vi "Arduino read multiple frequencies cristains filter.vi"(7 "main loop iteration number":i32, 9 "arduino addresses in":T2, 11 "arduinos on?":bool) -> (1 "arduino addresses out":T2, 2 "arduino frequencies out":T1, 3 "arduinos on":bool)   [LabVIEW 2014]
uses:
  <vilib>/Analysis/baseanly.llb/Mean (DBL).vi
  <vilib>/Analysis/NI_AALBase.lvlib
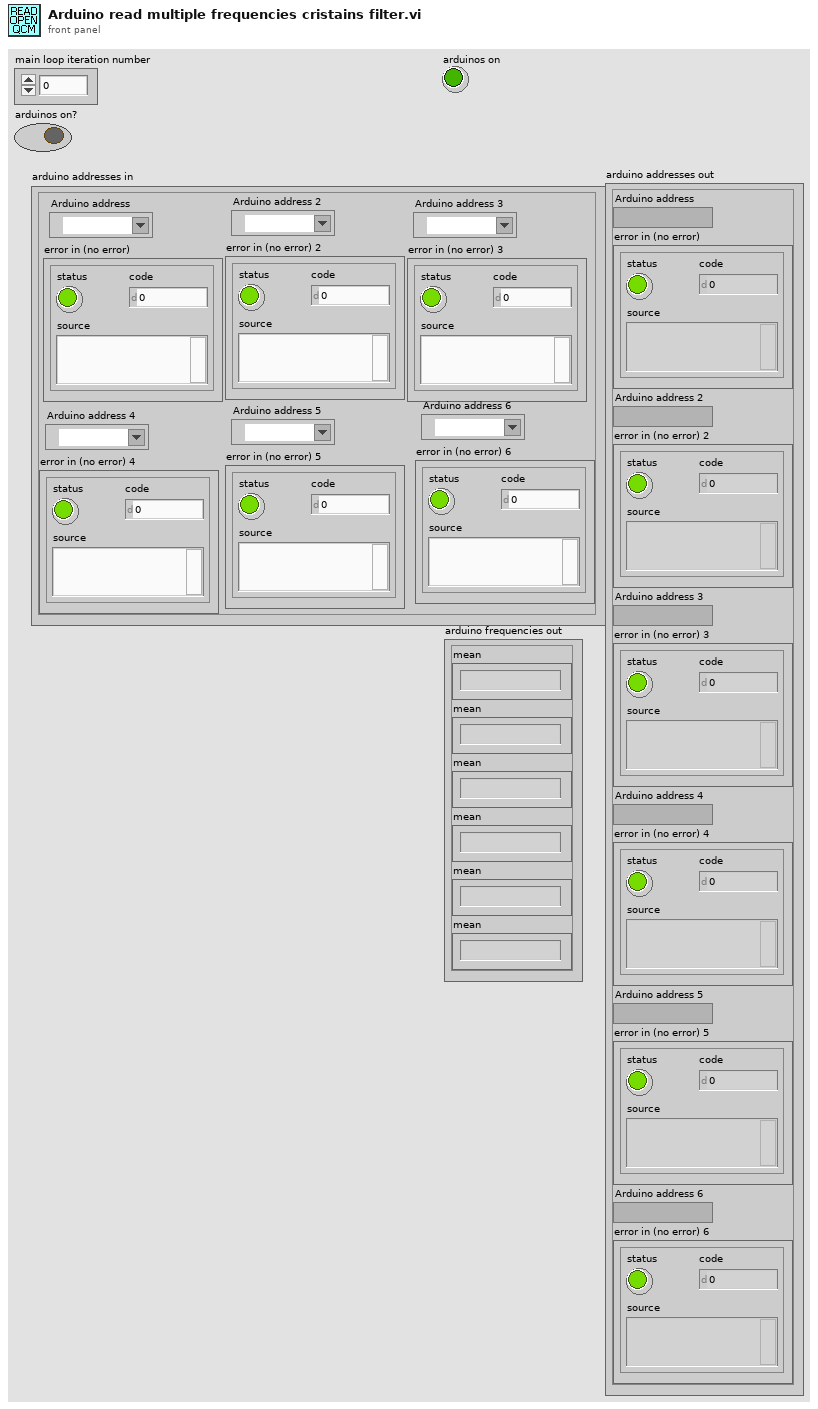
[diagram p1: front panel]
types:
  T1 = cluster{"mean":string, "mean":string, "mean":string, "mean":string, "mean":string, "mean":string}
  T2 = cluster{"Arduino address":refnum<visa-resource-name>, "error in (no error)":errorcluster, "Arduino address 2":refnum<visa-resource-name>, "error in (no error) 2":errorcluster, "Arduino address 3":refnum<visa-resource-name>, "error in (no error) 3":errorcluster, "Arduino address 4":refnum<visa-resource-name>, "error in (no error) 4":errorcluster, "Arduino address 5":refnum<visa-resource-name>, "error in (no error) 5":errorcluster, "Arduino address 6":refnum<visa-resource-name>, "error in (no error) 6":errorcluster}
  T3 = cluster{string, string, string, string, string, string}
  T4 = cluster{"Arduino address":refnum<visa-resource-name>, "error out":errorcluster, "Arduino address 2":refnum<visa-resource-name>, "error out":errorcluster, "Arduino address 3":refnum<visa-resource-name>, "error out":errorcluster, "Arduino address 4":refnum<visa-resource-name>, "error out":errorcluster, "Arduino address 5":refnum<visa-resource-name>, "error out":errorcluster, "Arduino address 6":refnum<visa-resource-name>, "error out":errorcluster}
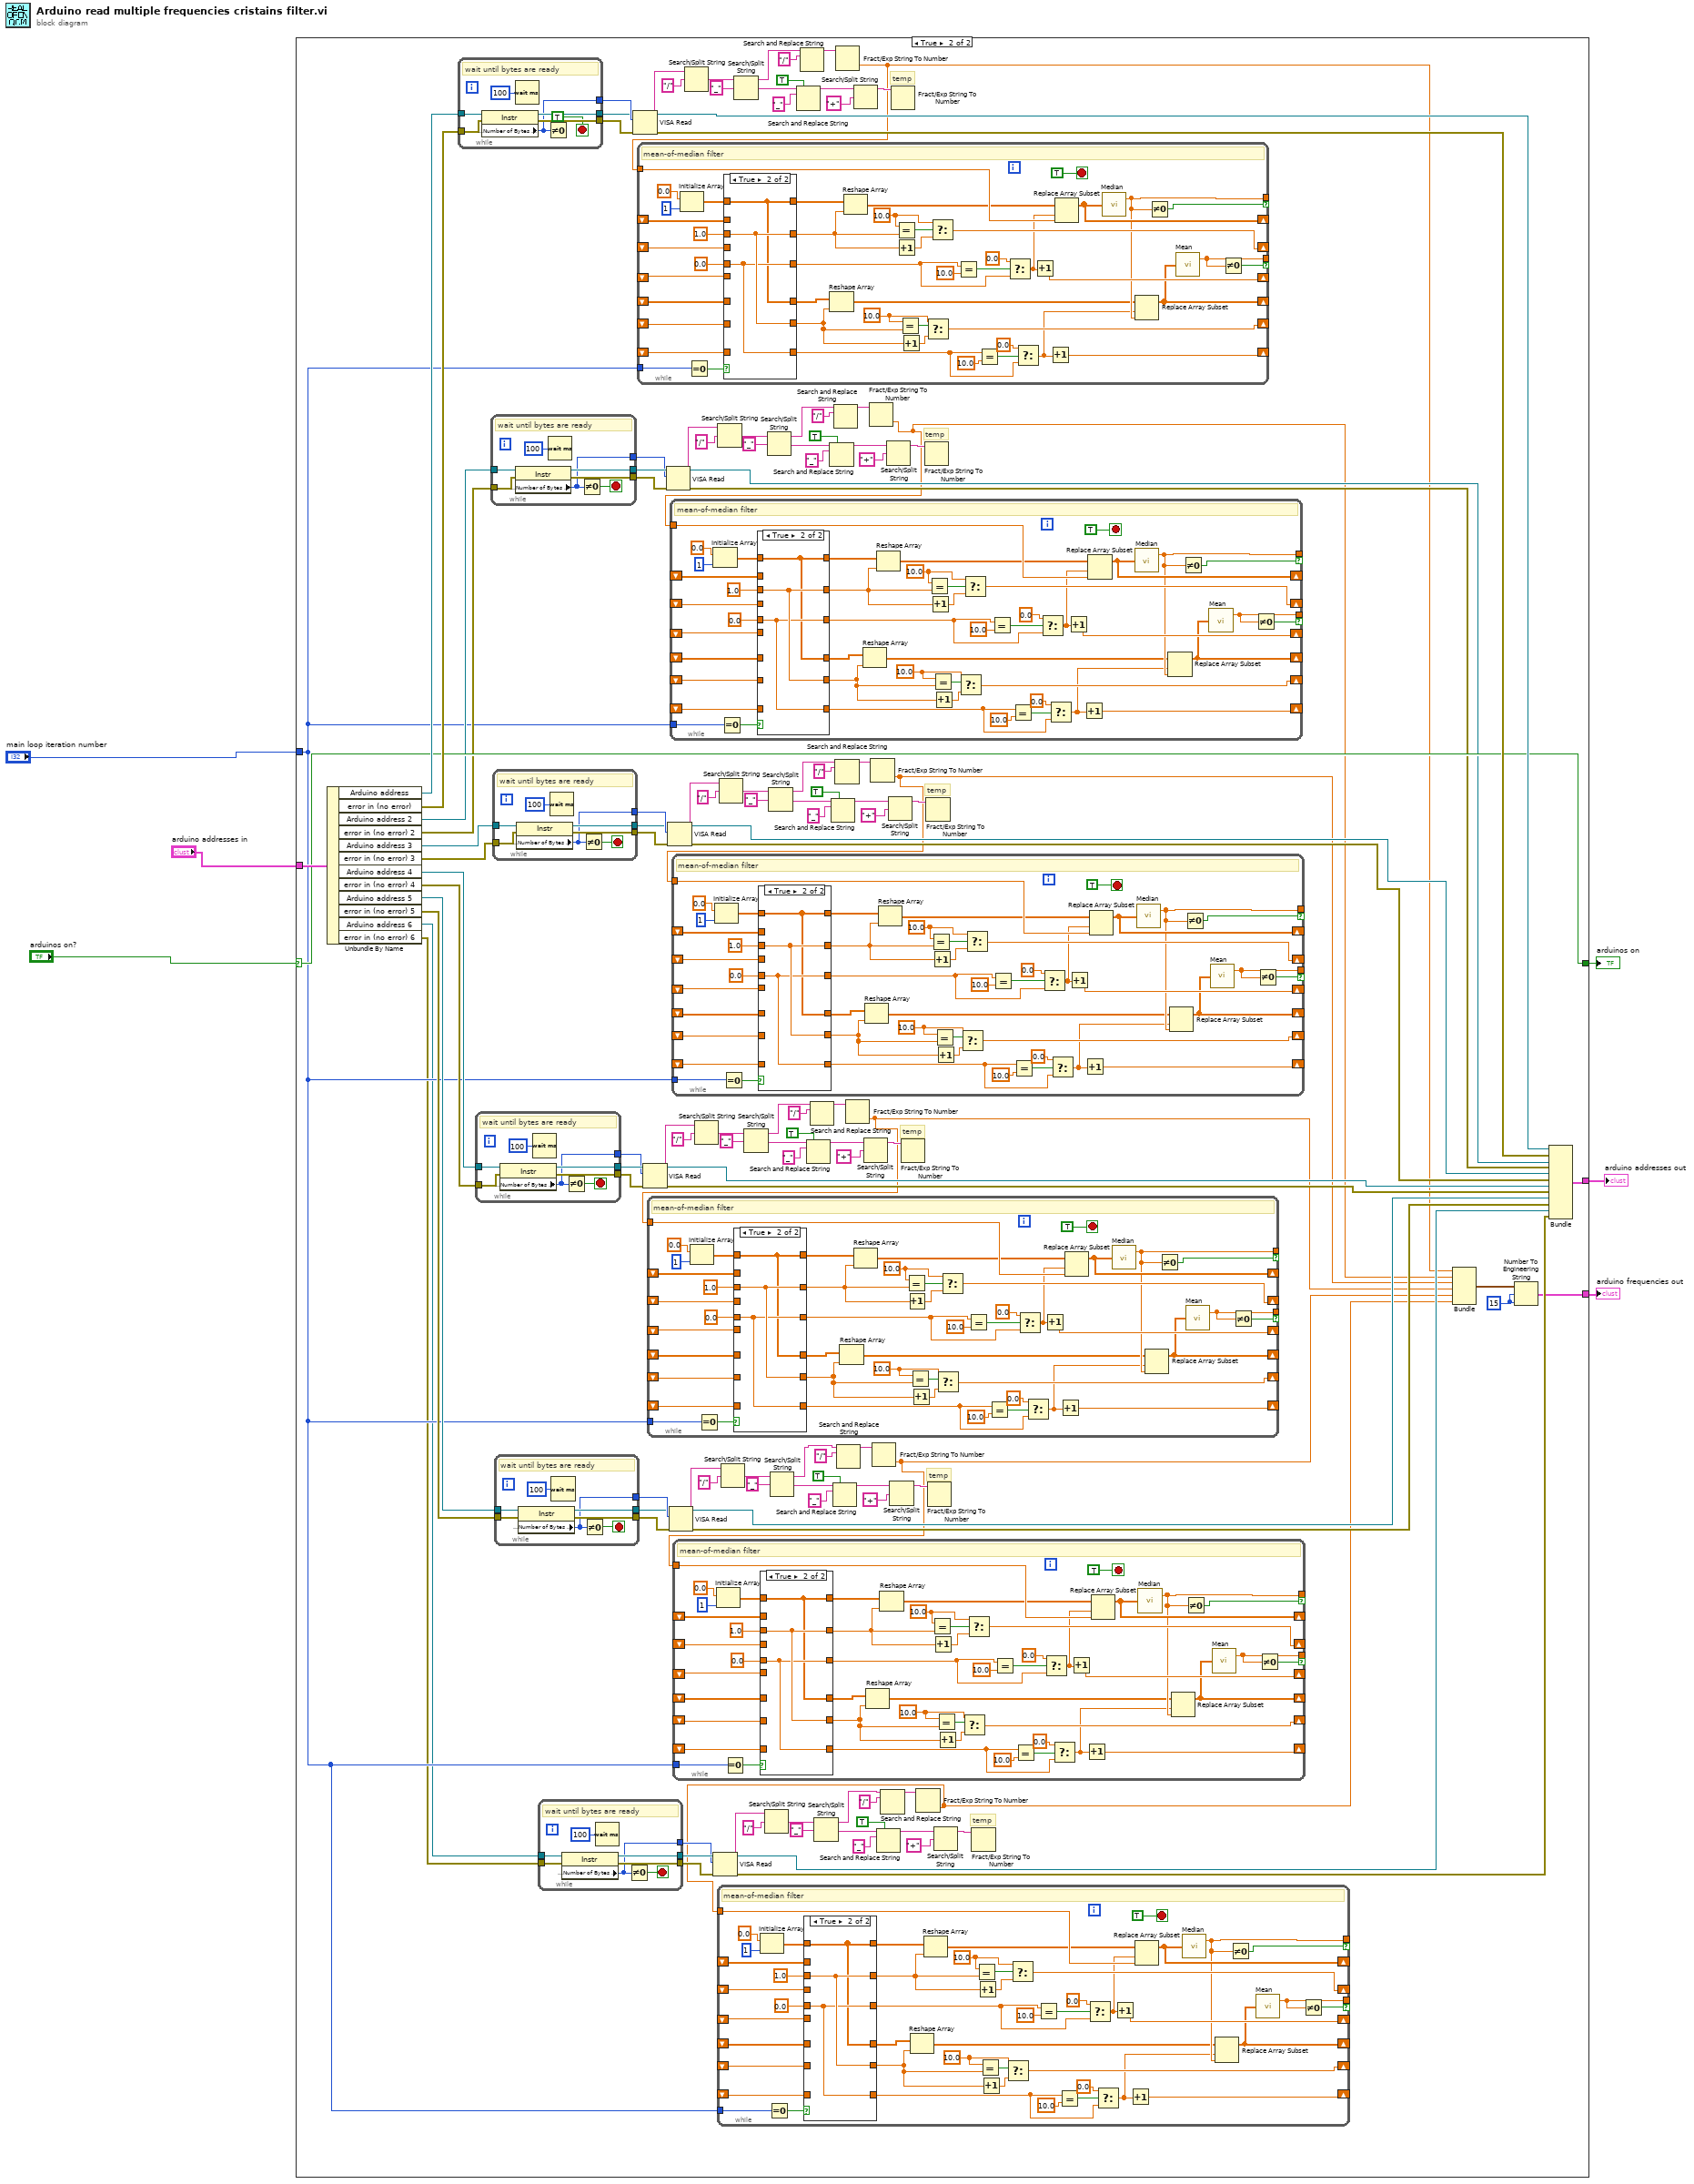
[diagram p0: block diagram]
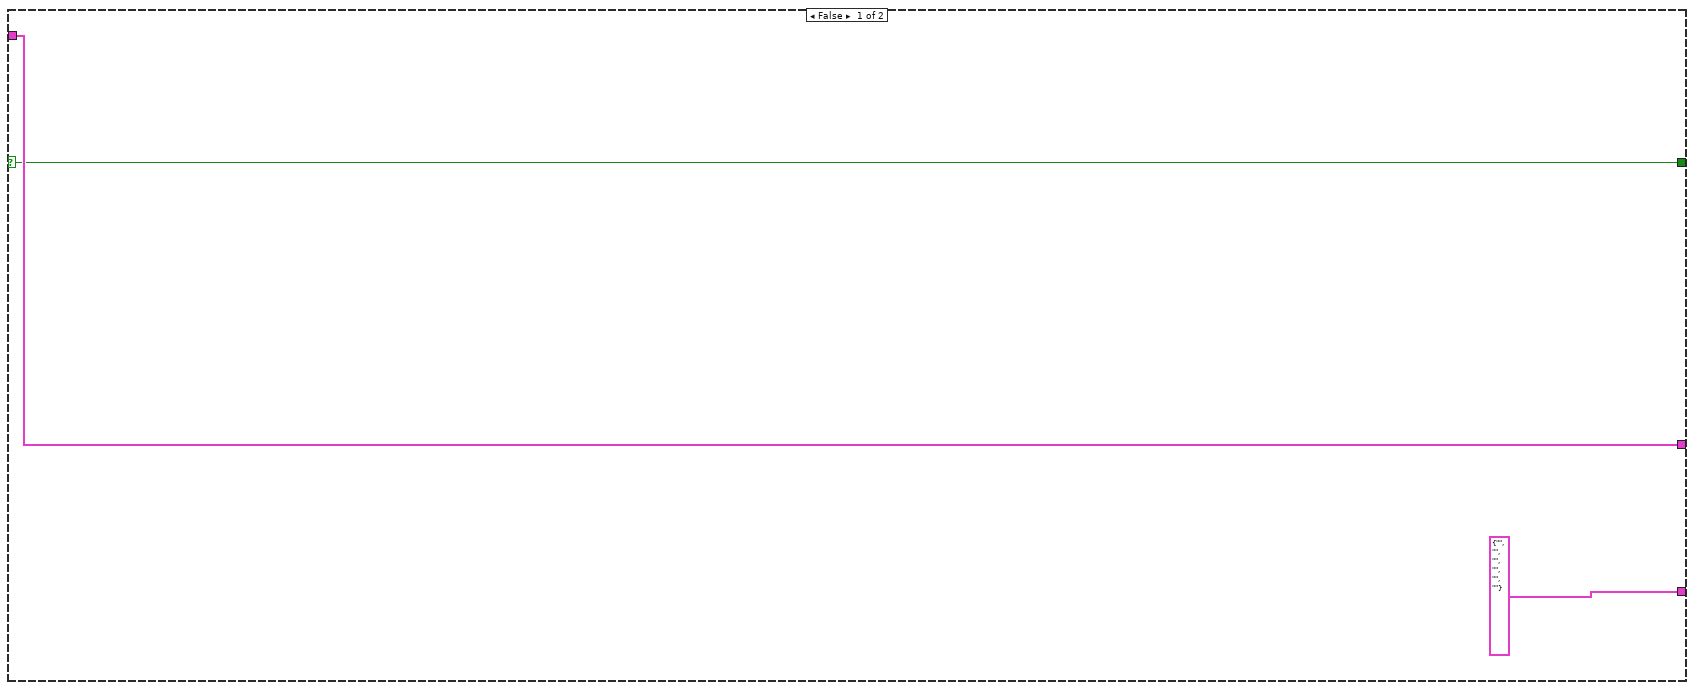
[diagram p2: hidden frame]
diagram:
  n1 = case shown="True" "arduinos on?" {
    selector: "arduinos on?" -> [w8 w120]
    tunnel: "main loop iteration number" -> [_ w25]
    tunnel: "arduino addresses in" -> [w9 w126]
    tunnel: [w9 w121] -> w2
    tunnel: [w8 w120] -> w3
    tunnel: [T1 {"mean"="", "mean"="", "mean"="", "mean"="", "mean"="", "mean"=""} w16] -> w1
    frame False {
    }
    frame True {
      w18 = i16 15 ("width (-)")
      # "temp"
      # "temp"
      # "temp"
      # "temp"
      # "temp"
      # "temp"
      n2 = Unbundle By Name(w126) -> ("Arduino address"=w125:refnum<visa-resource-name>, "error in (no error)"=w124:errorcluster, "Arduino address 2"=w103:refnum<visa-resource-name>, "error in (no error) 2"=w102:errorcluster, "Arduino address 3"=w83:refnum<visa-resource-name>, "error in (no error) 3"=w82:errorcluster, "Arduino address 4"=w63:refnum<visa-resource-name>, "error in (no error) 4"=w62:errorcluster, "Arduino address 5"=w45:refnum<visa-resource-name>, "error in (no error) 5"=w44:errorcluster, "Arduino address 6"=w24:refnum<visa-resource-name>, "error in (no error) 6"=w23:errorcluster)
      n3 = while {
        tunnel: w124 -> [w463]
        tunnel: w125 -> [w464]
        tunnel: [w462] -> w128
        tunnel: [w461] -> w127
        tunnel: [w460] -> w129
        stop <- TRUE stop-if-true
        # "wait until bytes are ready"
        n4 = property class="Instr"(reference=w464, error in=w463) -> (reference out=w461:refnum<visa-resource-name>, error out=w462:errorcluster, "Serial Settings:Number of Bytes at Serial Port"=w460:u32)
        n5 = Wait (ms)(milliseconds to wait=u32 100) -> ()  [unwired: 1 out]
        n6 = Not Equal To 0?(x=w460) -> ()  [unwired: 1 out]
      }
      n7 = while {
        tunnel: w62 -> [w274]
        tunnel: w63 -> [w275]
        tunnel: [w273] -> w78
        tunnel: [w272] -> w79
        tunnel: [w271] -> w77
        stop <- w269 stop-if-true
        # "wait until bytes are ready"
        n8 = property class="Instr"(reference=w275, error in=w274) -> (reference out=w272:refnum<visa-resource-name>, error out=w273:errorcluster, "Serial Settings:Number of Bytes at Serial Port"=w271:u32)
        n9 = Wait (ms)(milliseconds to wait=u32 100) -> ()  [unwired: 1 out]
        n10 = Not Equal To 0?(x=w271) -> (x != 0?=w269:bool)
      }
      n11 = while {
        tunnel: w102 -> [w400]
        tunnel: w103 -> [w401]
        tunnel: [w399] -> w118
        tunnel: [w398] -> w119
        tunnel: [w397] -> w117
        stop <- w395 stop-if-true
        # "wait until bytes are ready"
        n12 = property class="Instr"(reference=w401, error in=w400) -> (reference out=w398:refnum<visa-resource-name>, error out=w399:errorcluster, "Serial Settings:Number of Bytes at Serial Port"=w397:u32)
        n13 = Wait (ms)(milliseconds to wait=u32 100) -> ()  [unwired: 1 out]
        n14 = Not Equal To 0?(x=w397) -> (x != 0?=w395:bool)
      }
      n15 = while {
        tunnel: w82 -> [w337]
        tunnel: w83 -> [w338]
        tunnel: [w336] -> w85
        tunnel: [w335] -> w84
        tunnel: [w334] -> w86
        stop <- w332 stop-if-true
        # "wait until bytes are ready"
        n16 = property class="Instr"(reference=w338, error in=w337) -> (reference out=w335:refnum<visa-resource-name>, error out=w336:errorcluster, "Serial Settings:Number of Bytes at Serial Port"=w334:u32)
        n17 = Wait (ms)(milliseconds to wait=u32 100) -> ()  [unwired: 1 out]
        n18 = Not Equal To 0?(x=w334) -> (x != 0?=w332:bool)
      }
      n19 = while {
        tunnel: w45 -> [w212]
        tunnel: [w211] -> w47
        tunnel: [w210] -> w46
        tunnel: [w209] -> w48
        tunnel: w44 -> [w206]
        stop <- w207 stop-if-true
        # "wait until bytes are ready"
        n20 = property class="Instr"(reference=w212, error in=w206) -> (reference out=w210:refnum<visa-resource-name>, error out=w211:errorcluster, "Serial Settings:Number of Bytes at Serial Port"=w209:u32)
        n21 = Wait (ms)(milliseconds to wait=u32 100) -> ()  [unwired: 1 out]
        n22 = Not Equal To 0?(x=w209) -> (x != 0?=w207:bool)
      }
      n23 = while {
        tunnel: w24 -> [w149]
        tunnel: [w148] -> w40
        tunnel: [w147] -> w41
        tunnel: [w146] -> w39
        tunnel: w23 -> [w143]
        stop <- w144 stop-if-true
        # "wait until bytes are ready"
        n24 = property class="Instr"(reference=w149, error in=w143) -> (reference out=w147:refnum<visa-resource-name>, error out=w148:errorcluster, "Serial Settings:Number of Bytes at Serial Port"=w146:u32)
        n25 = Wait (ms)(milliseconds to wait=u32 100) -> ()  [unwired: 1 out]
        n26 = Not Equal To 0?(x=w146) -> (x != 0?=w144:bool)
      }
      n27 = VISA Read(VISA resource name=w127, byte count=w129, error in (no error)=w128) -> (VISA resource name out=w123:refnum<visa-resource-name>, read buffer=w142:string, error out=w122:errorcluster)  [unwired: 1 out]
      n28 = VISA Read(VISA resource name=w79, byte count=w77, error in (no error)=w78) -> (VISA resource name out=w61:refnum<visa-resource-name>, read buffer=w64:string, error out=w60:errorcluster)  [unwired: 1 out]
      n29 = VISA Read(VISA resource name=w119, byte count=w117, error in (no error)=w118) -> (VISA resource name out=w100:refnum<visa-resource-name>, read buffer=w104:string, error out=w101:errorcluster)  [unwired: 1 out]
      n30 = VISA Read(VISA resource name=w84, byte count=w86, error in (no error)=w85) -> (VISA resource name out=w81:refnum<visa-resource-name>, read buffer=w99:string, error out=w80:errorcluster)  [unwired: 1 out]
      n31 = VISA Read(VISA resource name=w46, byte count=w48, error in (no error)=w47) -> (VISA resource name out=w43:refnum<visa-resource-name>, read buffer=w59:string, error out=w42:errorcluster)  [unwired: 1 out]
      n32 = Search/Split String(string=w142, search string/char (-)="/") -> (match + rest of string=w135:string)  [unwired: 1 in, 2 out]
      n33 = Search/Split String(string=w64, search string/char (-)="/") -> (match + rest of string=w71:string)  [unwired: 1 in, 2 out]
      n34 = VISA Read(VISA resource name=w41, byte count=w39, error in (no error)=w40) -> (VISA resource name out=w20:refnum<visa-resource-name>, read buffer=w28:string, error out=w19:errorcluster)  [unwired: 1 out]
      n35 = Search/Split String(string=w104, search string/char (-)="/") -> (match + rest of string=w111:string)  [unwired: 1 in, 2 out]
      n36 = Search/Split String(string=w99, search string/char (-)="/") -> (match + rest of string=w92:string)  [unwired: 1 in, 2 out]
      n37 = Search/Split String(string=w59, search string/char (-)="/") -> (match + rest of string=w53:string)  [unwired: 1 in, 2 out]
      n38 = Search/Split String(string=w135, search string/char (-)="_") -> (substring before match=w141:string, match + rest of string=w136:string)  [unwired: 1 in, 1 out]
      n39 = Search/Split String(string=w71, search string/char (-)="_") -> (substring before match=w65:string, match + rest of string=w70:string)  [unwired: 1 in, 1 out]
      n40 = Search/Split String(string=w28, search string/char (-)="/") -> (match + rest of string=w34:string)  [unwired: 1 in, 2 out]
      n41 = Search/Split String(string=w111, search string/char (-)="_") -> (substring before match=w105:string, match + rest of string=w110:string)  [unwired: 1 in, 1 out]
      n42 = Search/Split String(string=w92, search string/char (-)="_") -> (substring before match=w98:string, match + rest of string=w93:string)  [unwired: 1 in, 1 out]
      n43 = Search/Split String(string=w53, search string/char (-)="_") -> (substring before match=w27:string, match + rest of string=w54:string)  [unwired: 1 in, 1 out]
      n44 = Search and Replace String(replace all?=TRUE ("replace all? (F)"), input string=w136, search string="_") -> (result string=w130:string)  [unwired: 5 in, 3 out]
      n45 = Search and Replace String(input string=w141, search string="/" ("replace string (\"\")")) -> (result string=w132:string)  [unwired: 6 in, 3 out]
      n46 = Search and Replace String(replace all?=TRUE ("replace all? (F)"), input string=w70, search string="_") -> (result string=w76:string)  [unwired: 5 in, 3 out]
      n47 = Search and Replace String(input string=w65, search string="/" ("replace string (\"\")")) -> (result string=w74:string)  [unwired: 6 in, 3 out]
      n48 = Search/Split String(string=w34, search string/char (-)="_") -> (substring before match=w22:string, match + rest of string=w33:string)  [unwired: 1 in, 1 out]
      n49 = Search and Replace String(replace all?=TRUE ("replace all? (F)"), input string=w110, search string="_") -> (result string=w116:string)  [unwired: 5 in, 3 out]
      n50 = Search and Replace String(replace all?=TRUE ("replace all? (F)"), input string=w93, search string="_") -> (result string=w87:string)  [unwired: 5 in, 3 out]
      n51 = Search and Replace String(replace all?=TRUE ("replace all? (F)"), input string=w54, search string="_") -> (result string=w49:string)  [unwired: 5 in, 3 out]
      n52 = Search and Replace String(input string=w105, search string="/" ("replace string (\"\")")) -> (result string=w114:string)  [unwired: 6 in, 3 out]
      n53 = Search and Replace String(input string=w98, search string="/" ("replace string (\"\")")) -> (result string=w89:string)  [unwired: 6 in, 3 out]
      n54 = Fract/Exp String To Number(string=w132) -> (number=w15:dbl)  [unwired: 3 in, 1 out]
      n55 = while {
        shift-right: [w503] -> _
        shift-left: _ -> [w481]
        shift-right: [w511] -> _
        shift-left: _ -> [w474]
        shift-right: [w500] -> _
        shift-left: _ -> [w471]
        shift-right: [w510] -> _
        shift-left: _ -> [w467]
        shift-right: [w509] -> _
        shift-left: _ -> [w478]
        tunnel: w15 -> [w506]
        tunnel: w25 -> [w483]
        tunnel: [w502] -> _ if=w505
        tunnel: [w499] -> _ if=w498
        shift-right: [w501] -> _
        shift-left: _ -> [w469]
        stop <- TRUE stop-if-true
        w484 = 10.0 ("t")
        w476 = 10.0 ("y")
        # "mean-of-median filter"
        n56 = Initialize Array(0.0 ("element"), 1 ("dimension size")) -> (w472:dbl[])
        n57 = Equal To 0?(x=w483) -> (x = 0?=w482:bool)
        n58 = case shown="True" w482 {
          tunnel: w472 -> [_ w518]
          tunnel: w481 -> [w517 _]
          tunnel: [w517 w518] -> w480
          tunnel: 1.0 ("t") -> [_ w520]
          tunnel: w478 -> [w516 _]
          tunnel: [w516 w520] -> w477
          tunnel: 0.0 ("t") -> [_ w519]
          tunnel: [w515 w519] -> w473
          tunnel: w474 -> [w515 _]
          tunnel: [w514 w518] -> w470
          tunnel: w471 -> [w514 _]
          tunnel: [w513 w520] -> w468
          tunnel: w469 -> [w513 _]
          tunnel: w467 -> [w512 _]
          tunnel: [w512 w519] -> w466
          frame False {
          }
          frame True {
          }
        }
        n59 = Reshape Array(w470, w468) -> (w465:dbl[])
        n60 = Reshape Array(w480, w477) -> (w491:dbl[])
        n61 = Equal?(x=w476, y=w477) -> (x = y?=w490:bool)
        n62 = Increment(x=w477) -> (x+1=w489:dbl)
        n63 = Equal?(x=w484, y=w468) -> (x = y?=w487:bool)
        n64 = Increment(x=w468) -> (x+1=w486:dbl)
        n65 = Select(t=w484, s=w487, f=w486) -> (s? t:f=w501:dbl)
        n66 = Select(t=w476, s=w490, f=w489) -> (s? t:f=w509:dbl)
        n67 = Equal?(x=w473, y=10.0) -> (x = y?=w497:bool)
        n68 = Equal?(x=w466, y=10.0) -> (x = y?=w494:bool)
        n69 = Select(t=0.0, s=w497, f=w473) -> (s? t:f=w485:dbl)
        n70 = Select(t=0.0, s=w494, f=w466) -> (s? t:f=w493:dbl)
        n71 = Increment(x=w485) -> (x+1=w511:dbl)
        n72 = Increment(x=w493) -> (x+1=w510:dbl)
        n73 = Replace Array Subset(array=w491, new element=w506, index=w485) -> (w503:dbl[])
        n74 = call <vilib>:"Median.vi"("X"=w503) -> ("median"=w499:dbl)  [unwired: 1 out]
        n75 = Replace Array Subset(array=w465, new element=w499, index=w493) -> (w500:dbl[])
        n76 = Not Equal To 0?(x=w499) -> (x != 0?=w498:bool)
        n77 = call-poly <vilib>:"Mean.vi"("X"=w500) -> ("mean"=w502:dbl)  [unwired: 1 out]
        n78 = Not Equal To 0?(x=w502) -> (x != 0?=w505:bool)
      }
      n79 = Search and Replace String(input string=w27, search string="/" ("replace string (\"\")")) -> (result string=w26:string)  [unwired: 6 in, 3 out]
      n80 = Fract/Exp String To Number(string=w74) -> (number=w12:dbl)  [unwired: 3 in, 1 out]
      n81 = while {
        shift-right: [w314] -> _
        shift-left: _ -> [w292]
        shift-right: [w322] -> _
        shift-left: _ -> [w285]
        shift-right: [w311] -> _
        shift-left: _ -> [w282]
        shift-right: [w321] -> _
        shift-left: _ -> [w278]
        shift-right: [w320] -> _
        shift-left: _ -> [w289]
        tunnel: w12 -> [w317]
        tunnel: w25 -> [w294]
        tunnel: [w313] -> _ if=w316
        tunnel: [w310] -> _ if=w309
        shift-right: [w312] -> _
        shift-left: _ -> [w280]
        stop <- TRUE stop-if-true
        w295 = 10.0 ("t")
        w287 = 10.0 ("y")
        # "mean-of-median filter"
        n82 = Initialize Array(0.0 ("element"), 1 ("dimension size")) -> (w283:dbl[])
        n83 = Equal To 0?(x=w294) -> (x = 0?=w293:bool)
        n84 = case shown="True" w293 {
          tunnel: w283 -> [_ w329]
          tunnel: w292 -> [w328 _]
          tunnel: [w328 w329] -> w291
          tunnel: 1.0 ("t") -> [_ w331]
          tunnel: w289 -> [w327 _]
          tunnel: [w327 w331] -> w288
          tunnel: 0.0 ("t") -> [_ w330]
          tunnel: [w326 w330] -> w284
          tunnel: w285 -> [w326 _]
          tunnel: [w325 w329] -> w281
          tunnel: w282 -> [w325 _]
          tunnel: [w324 w331] -> w279
          tunnel: w280 -> [w324 _]
          tunnel: w278 -> [w323 _]
          tunnel: [w323 w330] -> w277
          frame False {
          }
          frame True {
          }
        }
        n85 = Reshape Array(w281, w279) -> (w276:dbl[])
        n86 = Reshape Array(w291, w288) -> (w302:dbl[])
        n87 = Equal?(x=w287, y=w288) -> (x = y?=w301:bool)
        n88 = Increment(x=w288) -> (x+1=w300:dbl)
        n89 = Equal?(x=w295, y=w279) -> (x = y?=w298:bool)
        n90 = Increment(x=w279) -> (x+1=w297:dbl)
        n91 = Select(t=w295, s=w298, f=w297) -> (s? t:f=w312:dbl)
        n92 = Select(t=w287, s=w301, f=w300) -> (s? t:f=w320:dbl)
        n93 = Equal?(x=w284, y=10.0) -> (x = y?=w308:bool)
        n94 = Equal?(x=w277, y=10.0) -> (x = y?=w305:bool)
        n95 = Select(t=0.0, s=w308, f=w284) -> (s? t:f=w296:dbl)
        n96 = Select(t=0.0, s=w305, f=w277) -> (s? t:f=w304:dbl)
        n97 = Increment(x=w296) -> (x+1=w322:dbl)
        n98 = Increment(x=w304) -> (x+1=w321:dbl)
        n99 = Replace Array Subset(array=w302, new element=w317, index=w296) -> (w314:dbl[])
        n100 = call <vilib>:"Median.vi"("X"=w314) -> ("median"=w310:dbl)  [unwired: 1 out]
        n101 = Replace Array Subset(array=w276, new element=w310, index=w304) -> (w311:dbl[])
        n102 = Not Equal To 0?(x=w310) -> (x != 0?=w309:bool)
        n103 = call-poly <vilib>:"Mean.vi"("X"=w311) -> ("mean"=w313:dbl)  [unwired: 1 out]
        n104 = Not Equal To 0?(x=w313) -> (x != 0?=w316:bool)
      }
      n105 = Search/Split String(string=w130, search string/char (-)="+") -> (substring before match=w139:string)  [unwired: 1 in, 2 out]
      n106 = Search/Split String(string=w76, search string/char (-)="+") -> (substring before match=w67:string)  [unwired: 1 in, 2 out]
      n107 = Fract/Exp String To Number(string=w114) -> (number=w14:dbl)  [unwired: 3 in, 1 out]
      n108 = while {
        shift-right: [w440] -> _
        shift-left: _ -> [w418]
        shift-right: [w448] -> _
        shift-left: _ -> [w411]
        shift-right: [w437] -> _
        shift-left: _ -> [w408]
        shift-right: [w447] -> _
        shift-left: _ -> [w404]
        shift-right: [w446] -> _
        shift-left: _ -> [w415]
        tunnel: w14 -> [w443]
        tunnel: w25 -> [w420]
        tunnel: [w439] -> _ if=w442
        tunnel: [w436] -> _ if=w435
        shift-right: [w438] -> _
        shift-left: _ -> [w406]
        stop <- TRUE stop-if-true
        w421 = 10.0 ("t")
        w413 = 10.0 ("y")
        # "mean-of-median filter"
        n109 = Initialize Array(0.0 ("element"), 1 ("dimension size")) -> (w409:dbl[])
        n110 = Equal To 0?(x=w420) -> (x = 0?=w419:bool)
        n111 = case shown="True" w419 {
          tunnel: w409 -> [_ w455]
          tunnel: w418 -> [w454 _]
          tunnel: [w454 w455] -> w417
          tunnel: 1.0 ("t") -> [_ w457]
          tunnel: w415 -> [w453 _]
          tunnel: [w453 w457] -> w414
          tunnel: 0.0 ("t") -> [_ w456]
          tunnel: [w452 w456] -> w410
          tunnel: w411 -> [w452 _]
          tunnel: [w451 w455] -> w407
          tunnel: w408 -> [w451 _]
          tunnel: [w450 w457] -> w405
          tunnel: w406 -> [w450 _]
          tunnel: w404 -> [w449 _]
          tunnel: [w449 w456] -> w403
          frame False {
          }
          frame True {
          }
        }
        n112 = Reshape Array(w407, w405) -> (w402:dbl[])
        n113 = Reshape Array(w417, w414) -> (w428:dbl[])
        n114 = Equal?(x=w413, y=w414) -> (x = y?=w427:bool)
        n115 = Increment(x=w414) -> (x+1=w426:dbl)
        n116 = Equal?(x=w421, y=w405) -> (x = y?=w424:bool)
        n117 = Increment(x=w405) -> (x+1=w423:dbl)
        n118 = Select(t=w421, s=w424, f=w423) -> (s? t:f=w438:dbl)
        n119 = Select(t=w413, s=w427, f=w426) -> (s? t:f=w446:dbl)
        n120 = Equal?(x=w410, y=10.0) -> (x = y?=w434:bool)
        n121 = Equal?(x=w403, y=10.0) -> (x = y?=w431:bool)
        n122 = Select(t=0.0, s=w434, f=w410) -> (s? t:f=w422:dbl)
        n123 = Select(t=0.0, s=w431, f=w403) -> (s? t:f=w430:dbl)
        n124 = Increment(x=w422) -> (x+1=w448:dbl)
        n125 = Increment(x=w430) -> (x+1=w447:dbl)
        n126 = Replace Array Subset(array=w428, new element=w443, index=w422) -> (w440:dbl[])
        n127 = call <vilib>:"Median.vi"("X"=w440) -> ("median"=w436:dbl)  [unwired: 1 out]
        n128 = Replace Array Subset(array=w402, new element=w436, index=w430) -> (w437:dbl[])
        n129 = Not Equal To 0?(x=w436) -> (x != 0?=w435:bool)
        n130 = call-poly <vilib>:"Mean.vi"("X"=w437) -> ("mean"=w439:dbl)  [unwired: 1 out]
        n131 = Not Equal To 0?(x=w439) -> (x != 0?=w442:bool)
      }
      n132 = Fract/Exp String To Number(string=w89) -> (number=w13:dbl)  [unwired: 3 in, 1 out]
      n133 = while {
        shift-right: [w377] -> _
        shift-left: _ -> [w355]
        shift-right: [w385] -> _
        shift-left: _ -> [w348]
        shift-right: [w374] -> _
        shift-left: _ -> [w345]
        shift-right: [w384] -> _
        shift-left: _ -> [w341]
        shift-right: [w383] -> _
        shift-left: _ -> [w352]
        tunnel: w13 -> [w380]
        tunnel: w25 -> [w357]
        tunnel: [w376] -> _ if=w379
        tunnel: [w373] -> _ if=w372
        shift-right: [w375] -> _
        shift-left: _ -> [w343]
        stop <- TRUE stop-if-true
        w358 = 10.0 ("t")
        w350 = 10.0 ("y")
        # "mean-of-median filter"
        n134 = Initialize Array(0.0 ("element"), 1 ("dimension size")) -> (w346:dbl[])
        n135 = Equal To 0?(x=w357) -> (x = 0?=w356:bool)
        n136 = case shown="True" w356 {
          tunnel: w346 -> [_ w392]
          tunnel: w355 -> [w391 _]
          tunnel: [w391 w392] -> w354
          tunnel: 1.0 ("t") -> [_ w394]
          tunnel: w352 -> [w390 _]
          tunnel: [w390 w394] -> w351
          tunnel: 0.0 ("t") -> [_ w393]
          tunnel: [w389 w393] -> w347
          tunnel: w348 -> [w389 _]
          tunnel: [w388 w392] -> w344
          tunnel: w345 -> [w388 _]
          tunnel: [w387 w394] -> w342
          tunnel: w343 -> [w387 _]
          tunnel: w341 -> [w386 _]
          tunnel: [w386 w393] -> w340
          frame False {
          }
          frame True {
          }
        }
        n137 = Reshape Array(w344, w342) -> (w339:dbl[])
        n138 = Reshape Array(w354, w351) -> (w365:dbl[])
        n139 = Equal?(x=w350, y=w351) -> (x = y?=w364:bool)
        n140 = Increment(x=w351) -> (x+1=w363:dbl)
        n141 = Equal?(x=w358, y=w342) -> (x = y?=w361:bool)
        n142 = Increment(x=w342) -> (x+1=w360:dbl)
        n143 = Select(t=w358, s=w361, f=w360) -> (s? t:f=w375:dbl)
        n144 = Select(t=w350, s=w364, f=w363) -> (s? t:f=w383:dbl)
        n145 = Equal?(x=w347, y=10.0) -> (x = y?=w371:bool)
        n146 = Equal?(x=w340, y=10.0) -> (x = y?=w368:bool)
        n147 = Select(t=0.0, s=w371, f=w347) -> (s? t:f=w359:dbl)
        n148 = Select(t=0.0, s=w368, f=w340) -> (s? t:f=w367:dbl)
        n149 = Increment(x=w359) -> (x+1=w385:dbl)
        n150 = Increment(x=w367) -> (x+1=w384:dbl)
        n151 = Replace Array Subset(array=w365, new element=w380, index=w359) -> (w377:dbl[])
        n152 = call <vilib>:"Median.vi"("X"=w377) -> ("median"=w373:dbl)  [unwired: 1 out]
        n153 = Replace Array Subset(array=w339, new element=w373, index=w367) -> (w374:dbl[])
        n154 = Not Equal To 0?(x=w373) -> (x != 0?=w372:bool)
        n155 = call-poly <vilib>:"Mean.vi"("X"=w374) -> ("mean"=w376:dbl)  [unwired: 1 out]
        n156 = Not Equal To 0?(x=w376) -> (x != 0?=w379:bool)
      }
      n157 = Fract/Exp String To Number(string=w26) -> (number=w11:dbl)  [unwired: 3 in, 1 out]
      n158 = while {
        shift-right: [w251] -> _
        shift-left: _ -> [w229]
        shift-right: [w259] -> _
        shift-left: _ -> [w222]
        shift-right: [w248] -> _
        shift-left: _ -> [w219]
        shift-right: [w258] -> _
        shift-left: _ -> [w215]
        shift-right: [w257] -> _
        shift-left: _ -> [w226]
        tunnel: w11 -> [w254]
        tunnel: w25 -> [w231]
        tunnel: [w250] -> _ if=w253
        tunnel: [w247] -> _ if=w246
        shift-right: [w249] -> _
        shift-left: _ -> [w217]
        stop <- TRUE stop-if-true
        w232 = 10.0 ("t")
        w224 = 10.0 ("y")
        # "mean-of-median filter"
        n159 = Initialize Array(0.0 ("element"), 1 ("dimension size")) -> (w220:dbl[])
        n160 = Equal To 0?(x=w231) -> (x = 0?=w230:bool)
        n161 = case shown="True" w230 {
          tunnel: w220 -> [_ w266]
          tunnel: w229 -> [w265 _]
          tunnel: [w265 w266] -> w228
          tunnel: 1.0 ("t") -> [_ w268]
          tunnel: w226 -> [w264 _]
          tunnel: [w264 w268] -> w225
          tunnel: 0.0 ("t") -> [_ w267]
          tunnel: [w263 w267] -> w221
          tunnel: w222 -> [w263 _]
          tunnel: [w262 w266] -> w218
          tunnel: w219 -> [w262 _]
          tunnel: [w261 w268] -> w216
          tunnel: w217 -> [w261 _]
          tunnel: w215 -> [w260 _]
          tunnel: [w260 w267] -> w214
          frame False {
          }
          frame True {
          }
        }
        n162 = Reshape Array(w218, w216) -> (w213:dbl[])
        n163 = Reshape Array(w228, w225) -> (w239:dbl[])
        n164 = Equal?(x=w224, y=w225) -> (x = y?=w238:bool)
        n165 = Increment(x=w225) -> (x+1=w237:dbl)
        n166 = Equal?(x=w232, y=w216) -> (x = y?=w235:bool)
        n167 = Increment(x=w216) -> (x+1=w234:dbl)
        n168 = Select(t=w232, s=w235, f=w234) -> (s? t:f=w249:dbl)
        n169 = Select(t=w224, s=w238, f=w237) -> (s? t:f=w257:dbl)
        n170 = Equal?(x=w221, y=10.0) -> (x = y?=w245:bool)
        n171 = Equal?(x=w214, y=10.0) -> (x = y?=w242:bool)
        n172 = Select(t=0.0, s=w245, f=w221) -> (s? t:f=w233:dbl)
        n173 = Select(t=0.0, s=w242, f=w214) -> (s? t:f=w241:dbl)
        n174 = Increment(x=w233) -> (x+1=w259:dbl)
        n175 = Increment(x=w241) -> (x+1=w258:dbl)
        n176 = Replace Array Subset(array=w239, new element=w254, index=w233) -> (w251:dbl[])
        n177 = call <vilib>:"Median.vi"("X"=w251) -> ("median"=w247:dbl)  [unwired: 1 out]
        n178 = Replace Array Subset(array=w213, new element=w247, index=w241) -> (w248:dbl[])
        n179 = Not Equal To 0?(x=w247) -> (x != 0?=w246:bool)
        n180 = call-poly <vilib>:"Mean.vi"("X"=w248) -> ("mean"=w250:dbl)  [unwired: 1 out]
        n181 = Not Equal To 0?(x=w250) -> (x != 0?=w253:bool)
      }
      n182 = Search and Replace String(replace all?=TRUE ("replace all? (F)"), input string=w33, search string="_") -> (result string=w38:string)  [unwired: 5 in, 3 out]
      n183 = Search and Replace String(input string=w22, search string="/" ("replace string (\"\")")) -> (result string=w21:string)  [unwired: 6 in, 3 out]
      n184 = Search/Split String(string=w116, search string/char (-)="+") -> (substring before match=w107:string)  [unwired: 1 in, 2 out]
      n185 = Search/Split String(string=w87, search string/char (-)="+") -> (substring before match=w96:string)  [unwired: 1 in, 2 out]
      n186 = Search/Split String(string=w49, search string/char (-)="+") -> (substring before match=w57:string)  [unwired: 1 in, 2 out]
      n187 = Fract/Exp String To Number(string=w139) -> ()  [unwired: 3 in, 2 out]
      n188 = Fract/Exp String To Number(string=w67) -> ()  [unwired: 3 in, 2 out]
      n189 = Fract/Exp String To Number(string=w21) -> (number=w10:dbl)  [unwired: 3 in, 1 out]
      n190 = while {
        shift-right: [w188] -> _
        shift-left: _ -> [w166]
        shift-right: [w196] -> _
        shift-left: _ -> [w159]
        shift-right: [w185] -> _
        shift-left: _ -> [w156]
        shift-right: [w195] -> _
        shift-left: _ -> [w152]
        shift-right: [w194] -> _
        shift-left: _ -> [w163]
        tunnel: w10 -> [w191]
        tunnel: w25 -> [w168]
        tunnel: [w187] -> _ if=w190
        tunnel: [w184] -> _ if=w183
        shift-right: [w186] -> _
        shift-left: _ -> [w154]
        stop <- TRUE stop-if-true
        w169 = 10.0 ("t")
        w161 = 10.0 ("y")
        # "mean-of-median filter"
        n191 = Initialize Array(0.0 ("element"), 1 ("dimension size")) -> (w157:dbl[])
        n192 = Equal To 0?(x=w168) -> (x = 0?=w167:bool)
        n193 = case shown="True" w167 {
          tunnel: w157 -> [_ w203]
          tunnel: w166 -> [w202 _]
          tunnel: [w202 w203] -> w165
          tunnel: 1.0 ("t") -> [_ w205]
          tunnel: w163 -> [w201 _]
          tunnel: [w201 w205] -> w162
          tunnel: 0.0 ("t") -> [_ w204]
          tunnel: [w200 w204] -> w158
          tunnel: w159 -> [w200 _]
          tunnel: [w199 w203] -> w155
          tunnel: w156 -> [w199 _]
          tunnel: [w198 w205] -> w153
          tunnel: w154 -> [w198 _]
          tunnel: w152 -> [w197 _]
          tunnel: [w197 w204] -> w151
          frame False {
          }
          frame True {
          }
        }
        n194 = Reshape Array(w155, w153) -> (w150:dbl[])
        n195 = Reshape Array(w165, w162) -> (w176:dbl[])
        n196 = Equal?(x=w161, y=w162) -> (x = y?=w175:bool)
        n197 = Increment(x=w162) -> (x+1=w174:dbl)
        n198 = Equal?(x=w169, y=w153) -> (x = y?=w172:bool)
        n199 = Increment(x=w153) -> (x+1=w171:dbl)
        n200 = Select(t=w169, s=w172, f=w171) -> (s? t:f=w186:dbl)
        n201 = Select(t=w161, s=w175, f=w174) -> (s? t:f=w194:dbl)
        n202 = Equal?(x=w158, y=10.0) -> (x = y?=w182:bool)
        n203 = Equal?(x=w151, y=10.0) -> (x = y?=w179:bool)
        n204 = Select(t=0.0, s=w182, f=w158) -> (s? t:f=w170:dbl)
        n205 = Select(t=0.0, s=w179, f=w151) -> (s? t:f=w178:dbl)
        n206 = Increment(x=w170) -> (x+1=w196:dbl)
        n207 = Increment(x=w178) -> (x+1=w195:dbl)
        n208 = Replace Array Subset(array=w176, new element=w191, index=w170) -> (w188:dbl[])
        n209 = call <vilib>:"Median.vi"("X"=w188) -> ("median"=w184:dbl)  [unwired: 1 out]
        n210 = Replace Array Subset(array=w150, new element=w184, index=w178) -> (w185:dbl[])
        n211 = Not Equal To 0?(x=w184) -> (x != 0?=w183:bool)
        n212 = call-poly <vilib>:"Mean.vi"("X"=w185) -> ("mean"=w187:dbl)  [unwired: 1 out]
        n213 = Not Equal To 0?(x=w187) -> (x != 0?=w190:bool)
      }
      n214 = Fract/Exp String To Number(string=w107) -> ()  [unwired: 3 in, 2 out]
      n215 = Fract/Exp String To Number(string=w96) -> ()  [unwired: 3 in, 2 out]
      n216 = Fract/Exp String To Number(string=w57) -> ()  [unwired: 3 in, 2 out]
      n217 = Search/Split String(string=w38, search string/char (-)="+") -> (substring before match=w30:string)  [unwired: 1 in, 2 out]
      n218 = Fract/Exp String To Number(string=w30) -> ()  [unwired: 3 in, 2 out]
      n219 = Bundle(w15, w14, w13, w12, w11, w10) -> (w17:cluster{dbl, dbl, dbl, dbl, dbl, dbl})  [unwired: 1 in]
      n220 = Number To Engineering String(2:w18, 3:w18, 4:w17) -> (0:w16:T3)  [unwired: 1 in]
      n221 = Bundle("Arduino address"=w123, "error out"=w122, "Arduino address 2"=w100, "error out"=w101, "Arduino address 3"=w81, "error out"=w80, "Arduino address 4"=w61, "error out"=w60, "Arduino address 5"=w43, "error out"=w42, "Arduino address 6"=w20, "error out"=w19) -> (w121:T4)  [unwired: 1 in]
    }
  }
  "arduinos on" <- w3
  "arduino addresses out" <- w2
  "arduino frequencies out" <- w1
